vi "whileState.vi"(8 "error in (no error)":errorcluster, 10 "State Data in":refnum<class "data.lvclass">, 11 "state in":refnum<class "state.lvclass">) -> (0 "error out":errorcluster, 2 "State Data out":refnum<class "data.lvclass">, 3 "state out":refnum<class "state.lvclass">)   [LabVIEW 2020, in "eos.lvlib" / "state.lvclass"]
uses:
  state.lvclass
  data/data.lvclass
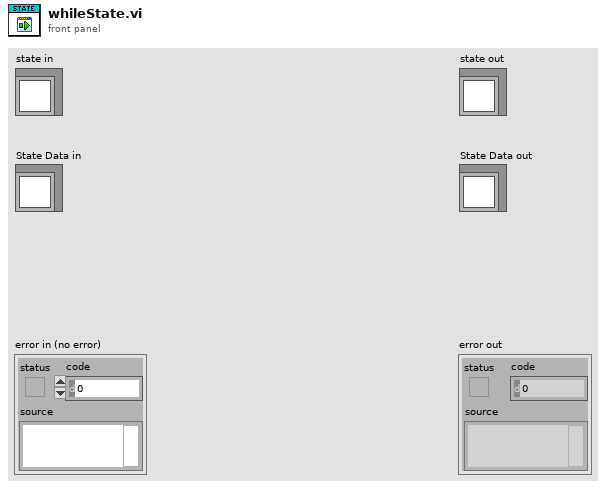
[diagram p1: front panel]
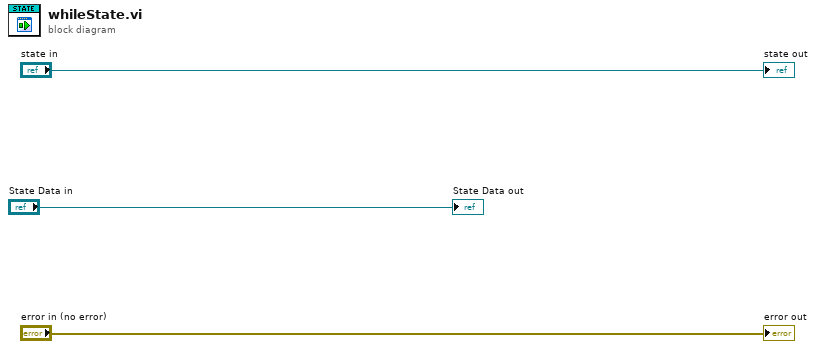
[diagram p0: block diagram]
diagram:
  "error out" <- "error in (no error)"
  "state out" <- "state in"
  "State Data out" <- "State Data in"
